vi "1D to 2D array.vi"(1 "1D Array Input":i16[](array[numeric]), 2 "Number of Columns":i32=16) -> (0 "2D Array Output":i16[][](array[numeric]))   [LabVIEW 2016]
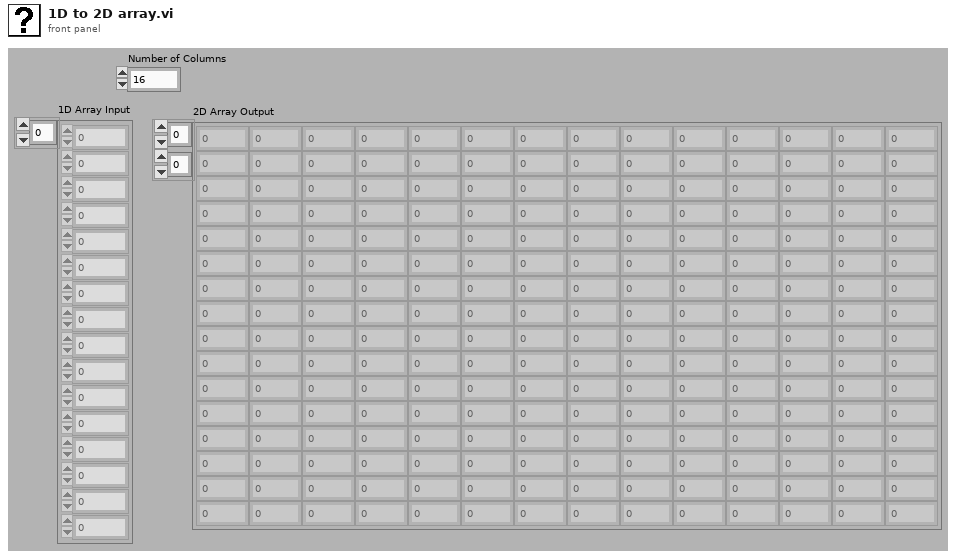
[diagram p1: front panel]
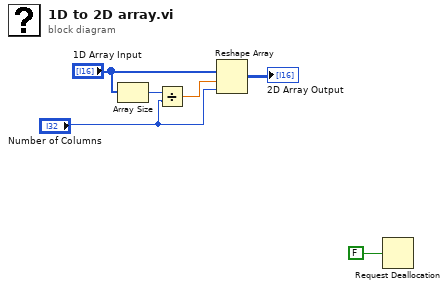
[diagram p0: block diagram]
diagram:
  n1 = Array Size(array="1D Array Input") -> (size(s)=w4:i32)
  n2 = Divide(x=w4, y="Number of Columns") -> (x/y=w3:dbl)
  n3 = Reshape Array("1D Array Input", w3, "Number of Columns") -> (→"2D Array Output":i16[][])
  n4 = Request Deallocation(FALSE ("flag")) -> ()
